vi "Testing - Go To Position.vi"() -> ()   [LabVIEW 2015]
uses:
  Position.ctl
  Type Defs/Direction Enum.ctl
  Square/Board Size.vi
  SubVIs/Read-Only Globals.vi
  Common.lvlib
  Type Defs/SB Type Defs.lvlib
panel:
  out "Direction":T1
  out "Position out":T2
  in  "Target Position":T2
  in  "My Position":T2
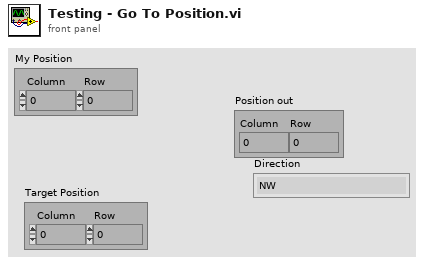
[diagram p1: front panel]
types:
  T1 = typedef "SB Type Defs.lvlib/Direction Enum.ctl" = enum16{"NW", "N", "NE", "E", "SE", "S", "SW", "W"}
  T2 = typedef "Common.lvlib/Position.ctl" = cluster{"Column":i32, "Row":i32}
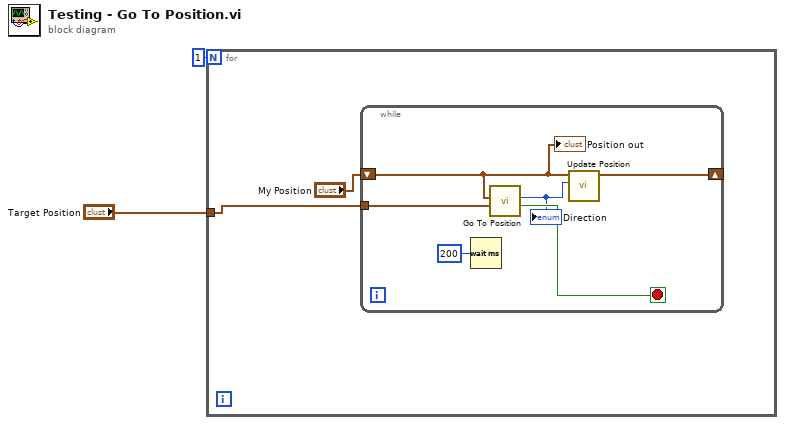
[diagram p0: block diagram]
diagram:
  n1 = for {
    N: 1 -> [_]
    tunnel: "Target Position" -> [w3]
    n2 = while {
      shift-right: [w9] -> _
      shift-left: "My Position" -> [w5]
      tunnel: w3 -> [w8]
      stop <- w10 stop-if-true
      n3 = Wait (ms)(milliseconds to wait=u32 200) -> ()  [unwired: 1 out]
      n4 = call "Go To Position.vi"("Target Position"=w8, "My Position"=w5) -> ("Arrived?"=w10:bool, "Direction"=w7:T1)  [unwired: 7 in, 1 out]
      "Direction" <- w7
      n5 = call "Update Position.vi"("Direction"=w7, "Position in"=w5) -> ("Position out"=w9:T2)  [unwired: 9 in]
      "Position out" <- w5
    }
  }
